vi "updateDisplacementsSettledArray.vi"(8 "error in (no error)":errorcluster, 10 "Distance Measured":dbl[unit]=1.0 min=1.0 max=300.0 format="%.1f", 11 "SystemController in":refnum<class "SystemController.lvclass">) -> (0 "error out":errorcluster, 2 "settledIsTrue":bool, 3 "SystemController out":refnum<class "SystemController.lvclass">)   [LabVIEW 2015, in "SystemController.lvclass"]
uses:
  SystemController.lvclass
  SystemController.lvclass/SystemController.ctl
  <vilib>/Analysis/NI_AALBase.lvlib
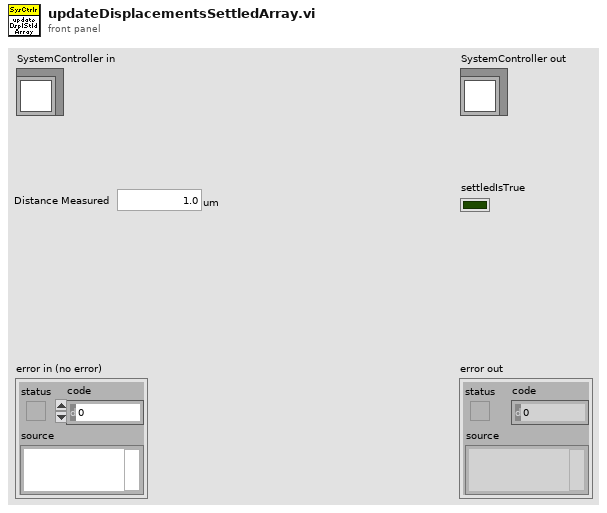
[diagram p1: front panel]
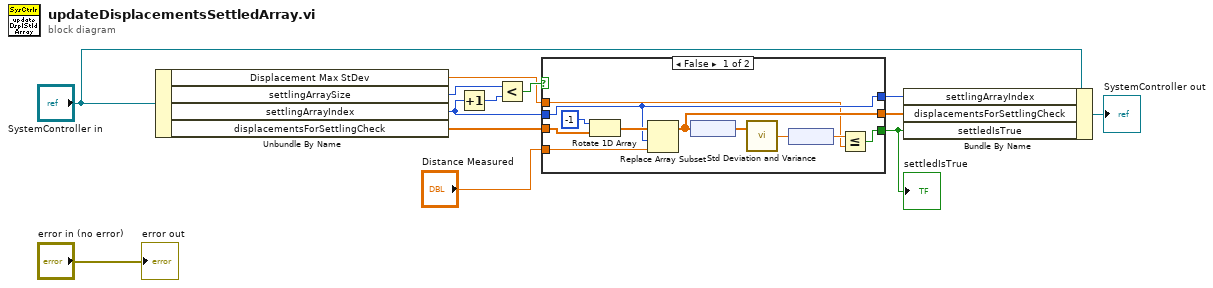
[diagram p0: block diagram]
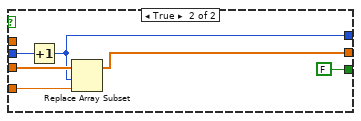
[diagram p2: hidden frame]
diagram:
  n1 = Unbundle By Name("SystemController in") -> ("Displacement Max StDev"=w2:dbl[unit], "settlingArraySize"=w10:i32, "settlingArrayIndex"=w4:i32, "displacementsForSettlingCheck"=w8:dbl[unit][])
  n2 = Increment(x=w4) -> (x+1=w9:i32)
  n3 = Less?(x=w10, y=w9) -> (x < y?=w5:bool)
  n4 = case shown="False" w5 {
    tunnel: w8 -> [w22 w30]
    tunnel: [w16 w28] -> w6
    tunnel: "Distance Measured" -> [w21 w29]
    tunnel: w4 -> [w20 w27]
    tunnel: [w20 w26] -> w3
    tunnel: w2 -> [w15 _]
    tunnel: [w14 FALSE] -> w1
    frame False {
      n5 = Rotate 1D Array(1:w22, 2:-1 ("n")) -> (0:w23:dbl[unit][])
      n6 = Replace Array Subset(array=w23, new element=w21, index=w20) -> (w16:dbl[unit][])
      n7 = node(w16) -> (w19:dbl[])
      n8 = call <vilib>:"Std Deviation and Variance.vi"("X"=w19) -> ("standard deviation"=w18:dbl)  [unwired: 1 in, 2 out]
      n9 = node(w18) -> (w17:dbl[unit])
      n10 = Less Or Equal?(x=w17, y=w15) -> (x <= y?=w14:bool)
    }
    frame True {
      n11 = Increment(x=w27) -> (x+1=w26:i32)
      n12 = Replace Array Subset(array=w30, new element=w29, index=w26) -> (w28:dbl[unit][])
    }
  }
  "settledIsTrue" <- w1
  n13 = Bundle By Name(cluster="SystemController in", "settlingArrayIndex"=w3, "displacementsForSettlingCheck"=w6, "settledIsTrue"=w1) -> (→"SystemController out":refnum<class "SystemController.lvclass">)
  "error out" <- "error in (no error)"
